vi "Teleop.vi"(10 "Match Info":T1={"Autonomous Elapsed Seconds"=0.0, "TeleOp Elapsed Seconds"=0.0, "Disabled Elapsed Seconds"=0.0, "Visited Autonomous"=FALSE, "Visited TeleOp"=FALSE, "Visited Disabled"=FALSE, "Autonomous Settings"={"Autonomous Style"=enum."Independent", "VI Refnum"=refnum}}, 11 "Call Context":T2) -> ()   [LabVIEW 2019]
doc: "This VI is called for each enabled TeleOp packet received from the DS. It is typically used to read from joysticks and other inputs and update I/O or setpoints for timed control loops. It should complete and return within 20 milliseconds or risk missing DS packets."
uses:
  <vilib>/Rock Robotics/WPI/DriverStation/WPI_DriverStationDerivedRobotMode.ctl
  <vilib>/Rock Robotics/WPI/DriverStation/WPI_DriverStationMatch Info.ctl
  <vilib>/Rock Robotics/WPI/Utilities/WPI_GetSetVariantRefNum.vi
  <vilib>/Rock Robotics/Network Tables/NT Write Boolean Array.vi
  <vilib>/Rock Robotics/Network Tables/NT Write Numeric Array.vi
  <vilib>/Rock Robotics/Network Tables/NT Write Boolean.vi
  <vilib>/Rock Robotics/Network Tables/NT Write Number.vi
  Framework/Robot Global Data.vi
panel:
  in  "DriveScale":dbl(slide)=0.7556179775280899 min=0.25 max=1.0 step=0.1 scale=0.25..1.0
  in  "Steering Scale":dbl(slide)=0.6418539325842696 min=0.25 max=1.0 step=0.1 scale=0.25..1.0
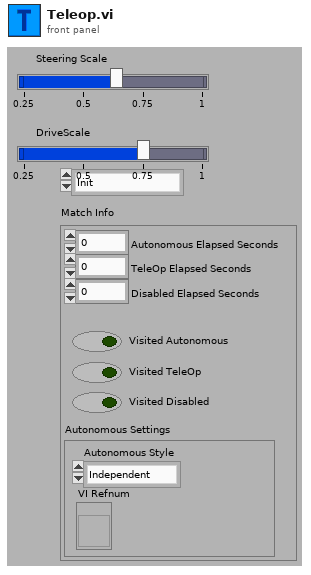
[diagram p1: front panel]
types:
  T1 = typedef "WPI_DriverStationMatch Info.ctl" = cluster{"Autonomous Elapsed Seconds":dbl, "TeleOp Elapsed Seconds":dbl, "Disabled Elapsed Seconds":dbl, "Visited Autonomous":bool, "Visited TeleOp":bool, "Visited Disabled":bool, "Autonomous Settings":cluster{"Autonomous Style":enum16{"Iterative", "Independent"}, "VI Refnum":refnum<vi>}}
  T2 = typedef "WPI_DriverStationDerivedRobotMode.ctl" = enum16{"Init", "Execute", "Stop"}
  T3 = typedef "WPI_JoystickDevRef.ctl" = cluster{"Device":T4}
  T4 = typedef "WPI_JoystickDeviceEnum.ctl" = enum16{"USB 0", "USB 1", "USB 2", "USB 3", "USB 4", "USB 5"}
  T5 = typedef "Command Status Info.ctl" = cluster{"Name":string, "Status":T6, "notifier out":T7}
  T6 = typedef "Completion Status.ctl" = enum16{"Successful", "Aborted", "Incomplete"}
  T7 = typedef "Completion Notifier.ctl" = refnum<notifier>
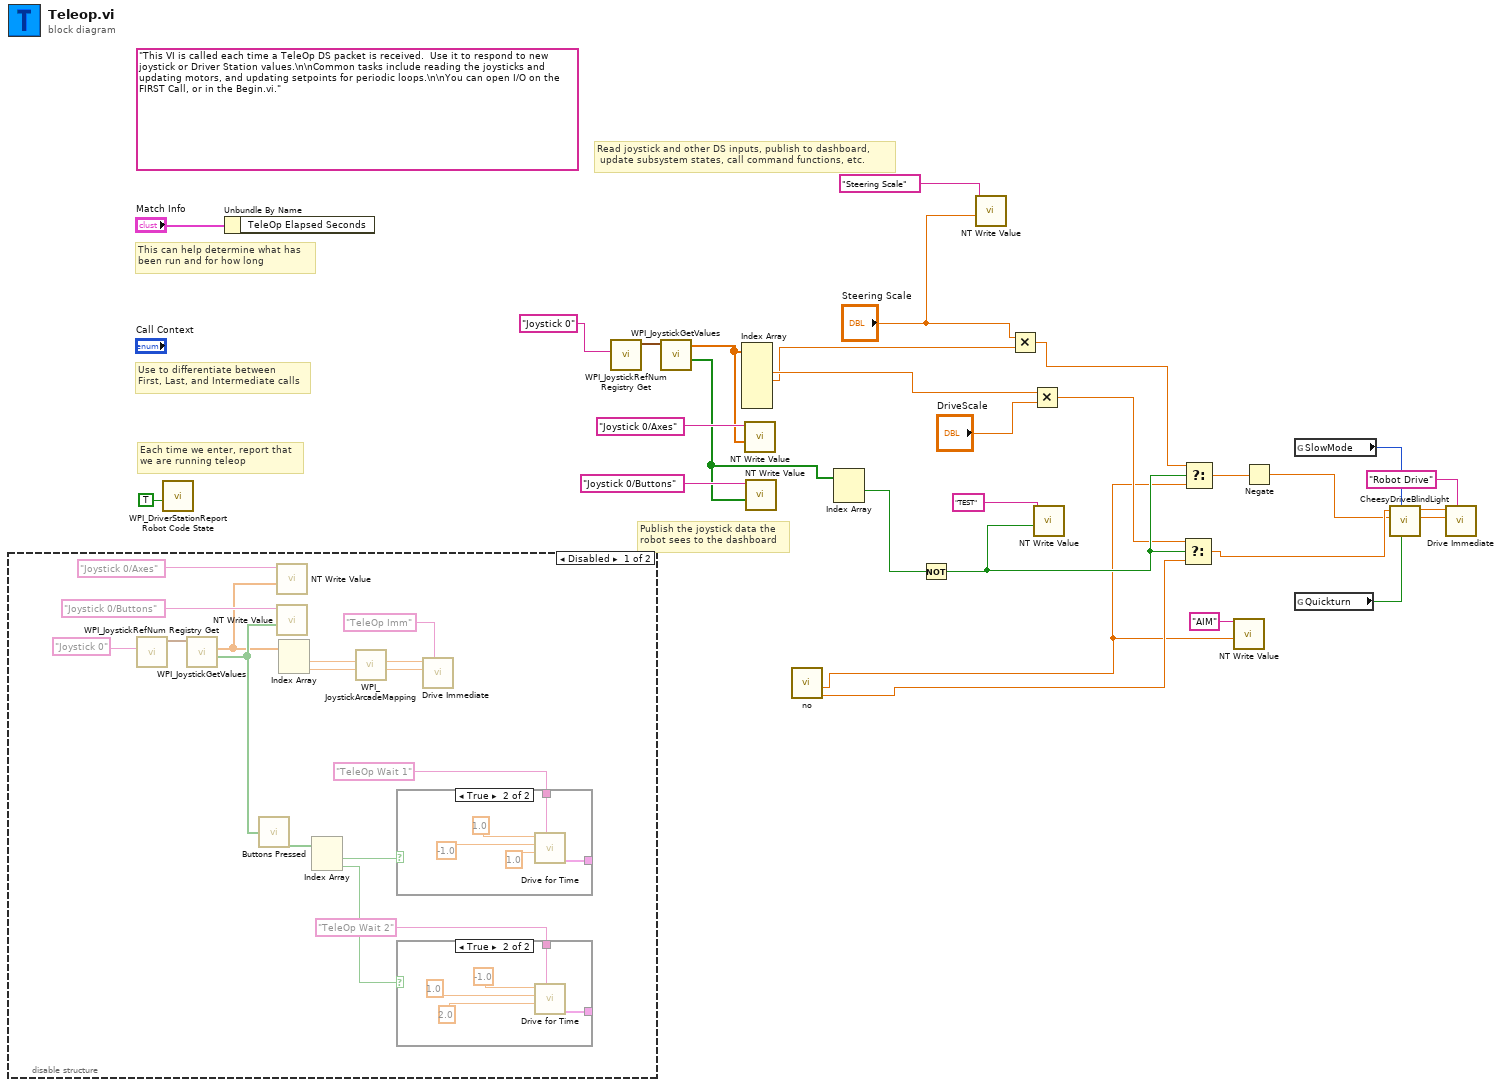
[diagram p0: block diagram]
diagram:
  (unwired) "This VI is called each time a TeleOp DS packet is received.  Use it to respond to new joystick or Driver Station values.\n\nCommon tasks include reading the joysticks and updating motors, and updating setpoints for periodic loops.\n\nYou can open I/O on the FIRST Call, or in the Begin.vi."
  # "Publish the joystick data the\nrobot sees to the dashboard"
  # "Read joystick and other DS inputs, publish to dashboard,\n update subsystem states, call command functions, etc."
  # "Each time we enter, report that\nwe are running teleop"
  # "Use to differentiate between\nFirst, Last, and Intermediate calls"
  # "This can help determine what has\nbeen run and for how long"
  n1 = disable-structure shown="Disabled" {
    frame Disabled {
      n2 = call <vilib>:"WPI_JoystickRefNum Registry Get.vi"("refnum name"="Joystick 0") -> ("JoystickDevRef"=w44:T3)  [unwired: 1 in, 9 out]
      n3 = call <vilib>:"WPI_JoystickGetValues.vi"("JoystickDevRef"=w44) -> ("Buttons"=w32:bool[], "Axes"=w31:dbl[])  [unwired: 6 in, 3 out]
      n4 = call "Buttons Pressed.vi"("Button Values"=w32) -> ("Button Presses"=w40:bool[])
      n5 = call-poly <vilib>:"NT Write Value.vi"("Numeric Array"=w31, "Name"="Joystick 0/Axes") -> ()  [unwired: 9 in, 1 out]
      n6 = call-poly <vilib>:"NT Write Value.vi"("Boolean Array"=w32, "Name"="Joystick 0/Buttons") -> ()  [unwired: 9 in, 1 out]
      n7 = Index Array(array=w31) -> (element #1=w35:dbl, element #2=w34:dbl)  [unwired: 2 in]
      n8 = Index Array(array=w40) -> (element #1=w39:bool, element #2=w38:bool)  [unwired: 2 in]
      n9 = call <vilib>:"WPI_JoystickArcadeMapping.vi"("Y axis value"=w34, "X axis value"=w35) -> ("Right Motor Value"=w36:dbl, "Left Motor Value"=w37:dbl)  [unwired: 8 in]
      n10 = case shown="True" w39 {
        tunnel: [_ w54] -> _
        tunnel: "TeleOp Wait 1" ("Description") -> [_ w53]
        frame False {
        }
        frame True {
          n11 = call "Drive for Time.vi"("Description"=w53, "Seconds"=1.0, "Right Speed"=-1.0, "Left Speed"=1.0) -> ("Command Info Out"=w54:T5)  [unwired: 7 in]
        }
      }
      n12 = case shown="True" w38 {
        tunnel: [_ w48] -> _
        tunnel: "TeleOp Wait 2" ("Description") -> [_ w47]
        frame False {
        }
        frame True {
          n13 = call "Drive for Time.vi"("Description"=w47, "Seconds"=2.0, "Right Speed"=1.0, "Left Speed"=-1.0) -> ("Command Info Out"=w48:T5)  [unwired: 7 in]
        }
      }
      n14 = call "Drive Immediate.vi"("Description"="TeleOp Imm", "Right Setpoint"=w36, "Left Setpoint"=w37) -> ()  [unwired: 8 in, 1 out]
    }
    frame Enabled {
    }
  }
  n15 = call <vilib>:"WPI_DriverStationReport Robot Code State.vi"("TeleOp"=TRUE ("Autonomous")) -> ()  [unwired: 10 in, 1 out]
  n16 = Unbundle By Name("Match Info") -> ()  [unwired: 1 out]
  n17 = call <vilib>:"WPI_JoystickRefNum Registry Get.vi"("refnum name"="Joystick 0") -> ("JoystickDevRef"=w26:T3)  [unwired: 1 in, 9 out]
  n18 = call <vilib>:"WPI_JoystickGetValues.vi"("JoystickDevRef"=w26) -> ("Buttons"=w22:bool[], "Axes"=w23:dbl[])  [unwired: 6 in, 3 out]
  n19 = Index Array(array=w23) -> (element #2=w16:dbl, element #3=w5:dbl)  [unwired: 6 in, 4 out]
  n20 = call-poly <vilib>:"NT Write Value.vi"("Numeric Array"=w23, "Name"="Joystick 0/Axes") -> ()  [unwired: 9 in, 1 out]
  n21 = call-poly <vilib>:"NT Write Value.vi"("Boolean Array"=w22, "Name"="Joystick 0/Buttons") -> ()  [unwired: 9 in, 1 out]
  n22 = call "no.vi"() -> ("DriveCommand"=w4:dbl, "SteerCommand"=w3:dbl)  [unwired: 9 in, 1 out]
  n23 = Index Array(array=w22) -> (element #1=w18:bool)  [unwired: 2 in, 1 out]
  n24 = Not(x=w18) -> (.not. x?=w19:bool)
  n25 = call-poly <vilib>:"NT Write Value.vi"("Numeric"="Steering Scale", "Name"="Steering Scale") -> ()  [unwired: 9 in, 1 out]
  n26 = Multiply(x="Steering Scale", y=w5) -> (x*y=w17:dbl)
  n27 = Multiply(x=w16, y="DriveScale") -> (x*y=w14:dbl)
  n28 = call-poly <vilib>:"NT Write Value.vi"("Boolean"=w19, "Name"="TEST") -> ()  [unwired: 9 in, 1 out]
  n29 = Select(t=w14, s=w19, f=w4) -> (s? t:f=w10:dbl)
  n30 = Select(t=w17, s=w19, f=w3) -> (s? t:f=w11:dbl)
  n31 = call-poly <vilib>:"NT Write Value.vi"("Numeric"=w3, "Name"="AIM") -> ()  [unwired: 9 in, 1 out]
  n32 = Negate(x=w11) -> (-x=w1:dbl)
  n33 = global read "Robot Global Data.vi" "SlowMode"() -> (w9:u32)
  n34 = global read "Robot Global Data.vi" "Quickturn"() -> (w2:bool)
  n35 = call "CheesyDriveBlindLight.vi"("Quickturn"=w2, "SlowMode"=w9, "Wheel"=w1, "Throttle"=w10) -> ("Right PWM"=w7:dbl, "Left PWM"=w8:dbl)  [unwired: 6 in]
  n36 = call "Drive Immediate.vi"("Description"="Robot Drive", "Right Setpoint"=w7, "Left Setpoint"=w8) -> ()  [unwired: 8 in, 1 out]
